vi "ObstacleBallRadius.vi"(9 "Goal":dbl[](array[numeric]), 10 "Initial State":dbl[](array[numeric]), 11 "ball":dbl[](array[numeric])) -> (2 "obstacle enemy radius":dbl)   [LabVIEW 2017]
uses:
  <vilib>/Analysis/_algsub.llb/Real Vector Norm.vi
  <vilib>/Analysis/NI_AALPro.lvlib
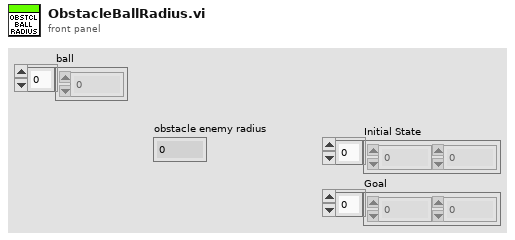
[diagram p1: front panel]
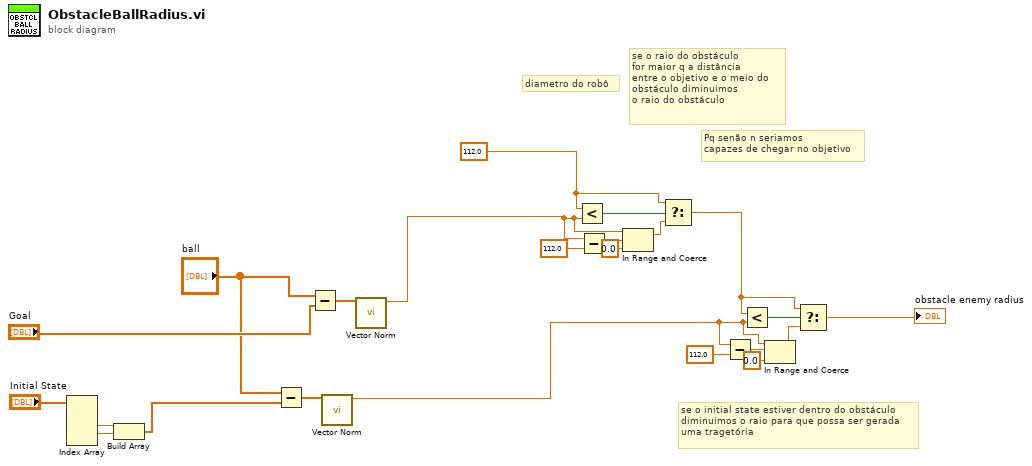
[diagram p0: block diagram]
diagram:
  w9 = 112.0 ("x")
  # "se o initial state estiver dentro do obstáculo\ndiminuimos o raio para que possa ser gerada\numa tragetória"
  # "diametro do robô"
  # "Pq senão n seriamos\ncapazes de chegar no objetivo"
  # "se o raio do obstáculo\nfor maior q a distância \nentre o objetivo e o meio do \nobstáculo diminuimos \no raio do obstáculo"
  n1 = Index Array(array="Initial State") -> (element #2=w13:dbl, element #3=w12:dbl)  [unwired: 4 in, 2 out]
  n2 = Build Array(w13, w12) -> (w11:dbl[])
  n3 = Subtract(x="ball", y=w11) -> (x-y=w20:dbl[])
  n4 = Subtract(x="ball", y="Goal") -> (x-y=w23:dbl[])
  n5 = call-poly <vilib>:"Vector Norm.vi"("Input Vector"=w20) -> ("norm"=w2:dbl)  [unwired: 9 in, 1 out]
  n6 = call-poly <vilib>:"Vector Norm.vi"("Input Vector"=w23) -> ("norm"=w7:dbl)  [unwired: 9 in, 1 out]
  n7 = Less?(x=w9, y=w7) -> (x < y?=w22:bool)
  n8 = Subtract(x=w7, y=112.0) -> (x-y=w8:dbl)
  n9 = In Range and Coerce(upper limit=w7, x=w8, lower limit=0.0) -> (coerced(x)=w5:dbl)  [unwired: 1 out]
  n10 = Select(t=w9, s=w22, f=w5) -> (s? t:f=w16:dbl)
  n11 = Subtract(x=w2, y=112.0) -> (x-y=w3:dbl)
  n12 = Less?(x=w16, y=w2) -> (x < y?=w18:bool)
  n13 = In Range and Coerce(upper limit=w2, x=w3, lower limit=0.0) -> (coerced(x)=w1:dbl)  [unwired: 1 out]
  n14 = Select(t=w16, s=w18, f=w1) -> (s? t:f=→"obstacle enemy radius":dbl)
